vi "Stop FP.vi"(8 "error in":errorcluster, 11 "PAS Control in":refnum<class "PAS Control.lvclass">) -> (0 "error out":errorcluster, 3 "PAS Control out":refnum<class "PAS Control.lvclass">)   [LabVIEW 2012, in "PAS Control.lvclass"]
uses:
  PAS Control.lvclass
  Reusable/GUI/GUI.lvclass
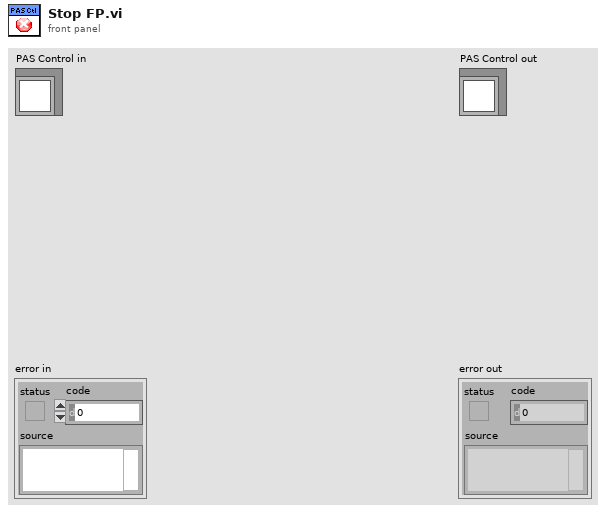
[diagram p1: front panel]
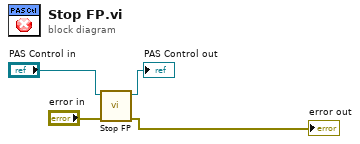
[diagram p0: block diagram]
diagram:
  n1 = call-parent "Stop FP.vi"("error in"="error in", "GUI in"="PAS Control in") -> ("error out"=→"error out":errorcluster, "GUI out"=→"PAS Control out":refnum<class "PAS Control.lvclass">)  [unwired: 8 in]
